vi "State_Machine.vi"(8 "error in (no error)":errorcluster caption="entrée d'erreur (pas d'erreur)", 11 "Get_Voltage en entrée":refnum<class "Nodon_Set_Switch_Type.lvclass">) -> (0 "error out":errorcluster caption="sortie d'erreur", 2 "Json_String":string, 3 "Get_Voltage en sortie":refnum<class "Nodon_Set_Switch_Type.lvclass">)   [LabVIEW 2020, in "Library Test.lvlib" / "Nodon_Set_Switch_Type.lvclass"]
uses:
  Nodon_Set_Switch_Type.lvclass
  C:/Users/ngarcin/OneDrive - Altyor/Standard TB/Class/Test/Test (Default)/Test (Default).lvclass
  C:/Users/ngarcin/OneDrive - Altyor/Standard TB/Class/Test/Nodon_Send_Command_UART/Nodon_Send_Command_UART.lvclass
  JSON API/JSON Value/Set from JSON string.vi
  JSON API/JSON Value/JSON Value.lvclass
  Nodon_Send_Command_UART.lvclass
  Nodon_Set_Switch_Type.lvclass/Nodon_Set_Switch_Type.ctl
  JSON API/Variant JSON/Variant JSON.lvlib
  JSON API/Get Polymorphic/JSON GetSet.lvlib
  Commun VI/Library Commun.lvlib
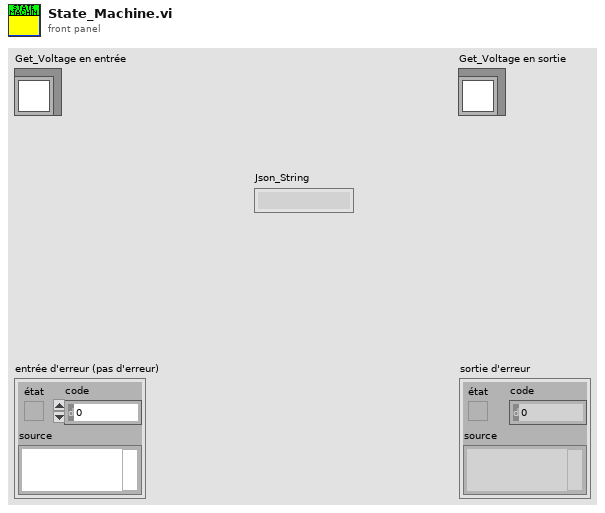
[diagram p1: front panel]
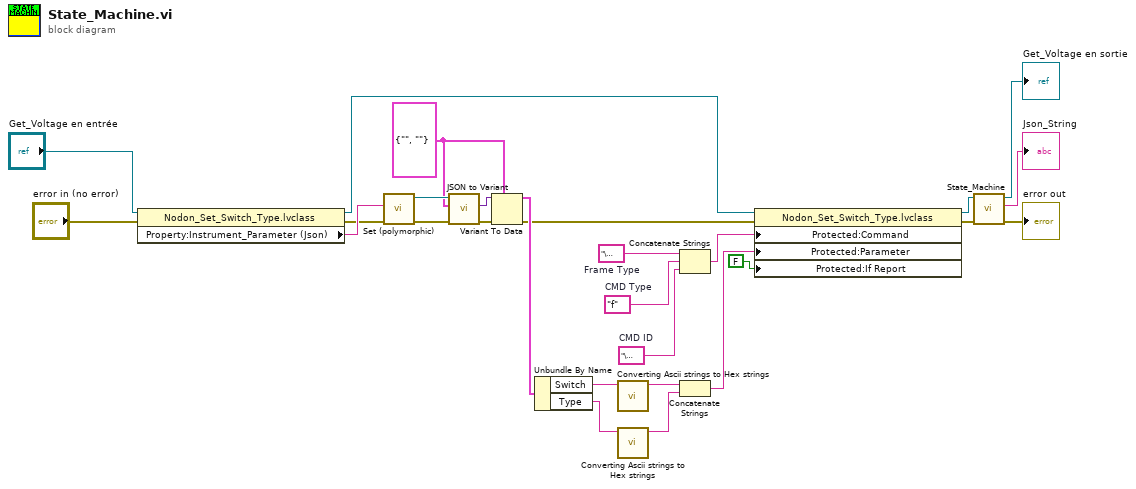
[diagram p0: block diagram]
diagram:
  w11 = cluster{"Switch":string, "Type":string} {"Switch"="", "Type"=""}
  w22 = "\u0000"  # Frame Type
  w21 = "\u0003"  # CMD ID
  w20 = "f"  # CMD Type
  n1 = property class="Nodon_Set_Switch_Type.lvclass"(reference="Get_Voltage en entrée", error in="error in (no error)") -> (reference out=w8:refnum<class "Nodon_Set_Switch_Type.lvclass">, error out=w13:errorcluster, "Property:Instrument_Parameter (Json)"=w14:string)
  n2 = call-poly "Set (polymorphic).vi"("error in (no error)"=w13, "JSON stream"=w14) -> ("error out"=w16:errorcluster, "JSON Value out"=w18:refnum<class "JSON Value.lvclass">)  [unwired: 7 in, 1 out]
  n3 = call "JSON to Variant.vi"("error in (no error)"=w16, "Variant (Data Type)"=w11, "JSON Value"=w18) -> ("error out"=w17:errorcluster, "Variant out"=w15:variant)  [unwired: 7 in]
  n4 = Variant To Data(error in=w17, type=w11, Variant=w15) -> (data=w10:cluster{"Switch":string, "Type":string}, error out=w5:errorcluster)
  n5 = Unbundle By Name(w10) -> ("Switch"=w6:string, "Type"=w4:string)
  n6 = call "Converting Ascii strings to Hex strings.vi"("result string"=w6) -> ("Chaîne"=w3:string)  [unwired: 10 in]
  n7 = call "Converting Ascii strings to Hex strings.vi"("result string"=w4) -> ("Chaîne"=w1:string)  [unwired: 10 in]
  n8 = Concatenate Strings(w22, w20, w21) -> (w19:string)
  n9 = Concatenate Strings(w3, w1) -> (w2:string)
  n10 = property class="Nodon_Set_Switch_Type.lvclass"(reference=w8, error in=w5, "Protected:Command"=w19, "Protected:Parameter"=w2, "Protected:If Report"=FALSE ("If Report")) -> (reference out=w24:refnum<class "Nodon_Set_Switch_Type.lvclass">, error out=w23:errorcluster)
  n11 = call-parent "State_Machine.vi"("error in (no error)"=w23, "Send_Frame en entrée"=w24) -> ("error out"=→"error out":errorcluster, "Json_String"=→"Json_String":string, "Send_Frame en sortie"=→"Get_Voltage en sortie":refnum<class "Nodon_Set_Switch_Type.lvclass">)  [unwired: 7 in]
